vi "Spline 보간 조향각계산.vi"() -> (0 "Steer Angle":dbl, 1 "부분행렬":T1)   [LabVIEW 2016]
uses:
  <vilib>/Analysis/Matrix/Datatypes/RealMatrix.ctl
  <vilib>/imath/engines/lvmath2/RunTimeEngine/Managers/WorkSpace/UID Generator.vi
  <vilib>/Analysis/Matrix/Numeric/Conversions/Matrix To Array - RM.vi
  <vilib>/imath/engines/lvmath2/RunTimeEngine/IndexRead/NIMS M(S,S).vi
  <instcachedir>/0/NIMS M(S,S)_AC51E74150A542F7991B9634C66F3096.lvgen/NIMS M(S,S)_AC51E74150A542F7991B9634C66F3096_000.vi
  <vilib>/imathl/engines/lvmath/Functions/Error Handling/Create Error.vi
  <vilib>/imath/engines/lvmath2/RunTimeEngine/RunTimeType/NIMS_RunTimeType_From StrictType (excl LVString).vi
  <instcachedir>/0/NIMS_RunTimeType_From StrictType (excl LVString)_BBF44FB49F834B71AF7A14CCEDF8BECD.lvgen/NIMS_RunTimeType_From StrictType (excl LVString)_BBF44FB49F834B71AF7A14CCEDF8BECD_000.vi
  <vilib>/imath/engines/lvmath2/RunTimeEngine/LocalVariableDefStatement/MC_LocalVariableDefStatement_Display.vi
  <vilib>/imath/engines/lvmath2/RunTimeSupport/NIMS_Complex To Real.vi
  <instcachedir>/0/NIMS_Complex To Real_A9DD49CC305F495FA24B9F5762C73A31.lvgen/NIMS_Complex To Real_A9DD49CC305F495FA24B9F5762C73A31_001.vi
  <vilib>/imath/engines/lvmath2/RunTimeEngine/BuiltInFunctions/rad_to_deg/NIMS_rad_to_deg.vi
  <instcachedir>/0/NIMS_rad_to_deg_A39AFCDDC8C049FCADAAB7FC30B9F5AA.lvgen/NIMS_rad_to_deg_A39AFCDDC8C049FCADAAB7FC30B9F5AA_001.vi
  <vilib>/imath/engines/lvmath2/RunTimeEngine/Managers/SymbolTable/Clear UID.vi
  <vilib>/imath/engines/lvmath2/RunTimeEngine/NodeEndStatement/NIMS_NodeEndStatement_Output.vi
  <instcachedir>/0/NIMS_NodeEndStatement_Output_53EC0D466D134D7ABD903AC30B43404B.lvgen/NIMS_NodeEndStatement_Output_53EC0D466D134D7ABD903AC30B43404B_001.vi
  <vilib>/imath/engines/lvmath2/RunTimeEngine/ErrorHandling/NIMS_Finalize Error.vi
  <vilib>/Analysis/NI_AALPro.lvlib
  <vilib>/Analysis/Matrix/NI_Matrix.lvlib
  <vilib>/imath/engines/lvmath2/RunTimeEngine/Managers/SymbolTable/NIMS_WorkSpace.lvlib
panel:
  in  "Lane Center":dbl[][](array[numeric]) format="%0.3f"
  out "Interpolated Data (X,Y)":dbl[][](array[numeric]) format="%0.2f"
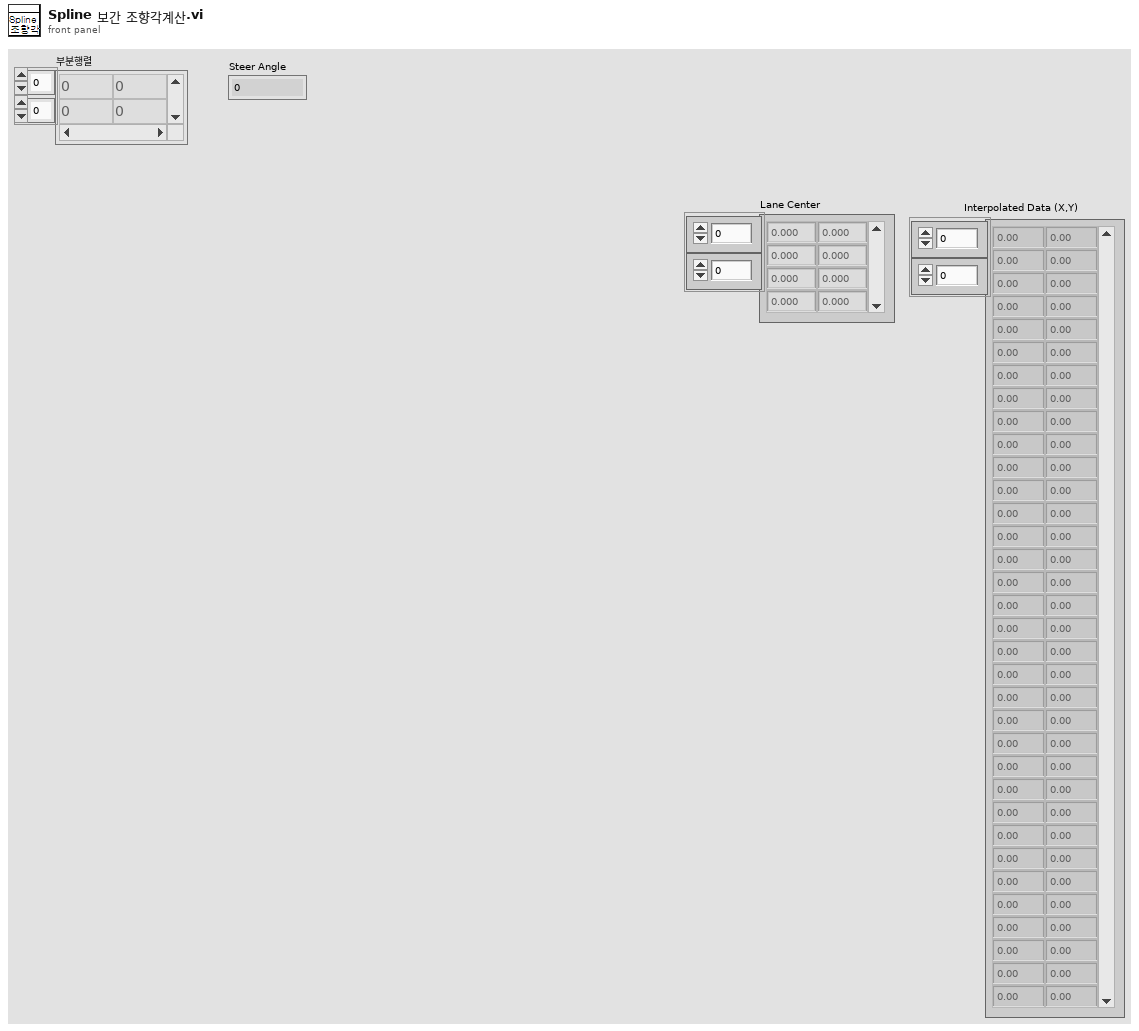
[diagram p1: front panel]
types:
  T1 = typedef "NI_Matrix.lvlib/RealMatrix.ctl" = dbl[][]
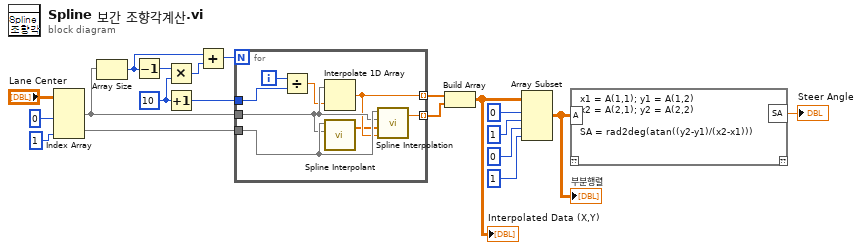
[diagram p0: block diagram]
diagram:
  w19 = 10 ("Interpolation factor (n)")
  n1 = Index Array(array="Lane Center", index (col) #1=0, index (col) #2=1 ("index (col)")) -> (element #1=w17:dbl[], element #2=w10:dbl[])  [unwired: 2 in]
  n2 = Array Size(array=w17) -> (size(s)=w13:i32)
  n3 = Decrement(x=w13) -> (x-1=w16:i32)
  n4 = Multiply(x=w16, y=w19) -> (x*y=w14:i32)
  n5 = Increment(x=w19) -> (x+1=w15:i32)
  n6 = Add(x=w13, y=w14) -> (x+y=w12:i32)
  n7 = for {
    N: w12 -> [_]
    tunnel: w10 -> [w28]
    tunnel: w17 -> [w24]
    tunnel: w15 -> [w26]
    tunnel: [w25] -> w8 mode=indexing
    tunnel: [w23] -> w9 mode=indexing
    i -> [w27]
    n8 = Divide(x=w27, y=w26) -> (x/y=w22:dbl)
    n9 = Interpolate 1D Array(1:w22, 2:w24) -> (0:w23:dbl)
    n10 = call <vilib>:"Spline Interpolant.vi"("X"=w24, "Y"=w28) -> ("Interpolant"=w21:dbl[])  [unwired: 2 in, 1 out]
    n11 = call <vilib>:"Spline Interpolation.vi"("x value"=w23, "Interpolant"=w21, "X"=w24, "Y"=w28) -> ("interpolation value"=w25:dbl)  [unwired: 1 out]
  }
  n12 = Build Array(w9, w8) -> (w7:T1)
  "Interpolated Data (X,Y)" <- w7
  n13 = Array Subset(array=w7, index (row)=0 ("행 1"), length (row)=1 ("행 N"), index (col)=0 ("열 1"), length (col)=1 ("열 N")) -> (w2:T1)
  "부분행렬" <- w2
  n14 = mathscript code="x1 = A(1,1); y1 = A(1,2)\nx2 = A(2,1); y2 = A(2,2)\n\nSA = rad2deg(atan((y2-y1)/(x2-x1)))"("A"=w2) -> ("SA"=→"Steer Angle":dbl)  [unwired: 1 in, 1 out]
